vi "Error Channels Read Single.vi"(8 "error in":errorcluster, 9 "Channel Index":i32=1, 11 "Error Channels In":refnum<class "Error Channels.lvclass">) -> (0 "error out":errorcluster, 1 "Changed or First Call?":bool, 2 "Error Acknowledge Channels ACT":bool, 3 "Error Channels Out":refnum<class "Error Channels.lvclass">)   [LabVIEW 2023, in "Error Channels.lvclass"]
uses:
  Error Channels.lvclass
  Error Channels.lvclass/Error Channels.ctl
  <vilib>/ADAS Replay HIL/Channels/Tag Wrapper/Polymorphic/Read Channel (Boolean).vi
  fe5b2b55-f13d-4754-bc7f-45dbc12555c6.vi
  <vilib>/ADAS Replay HIL/Channels/Tag Wrapper/Polymorphic/Read Channel (Boolean).vi/b2f764de-0c1e-4784-a155-687fc995a684.vi
  <vilib>/ADAS Replay HIL/Channels/Tag Wrapper/Polymorphic/Read Channel (Boolean).vi/b2f764de-0c1e-4784-a155-687fc995a684.vi/c28b0ead-42ad-4072-80a2-aca7f2bd7ce3.vi
  <vilib>/ADAS Replay HIL/Channels/Tag Wrapper/Polymorphic/Read Channel (Boolean).vi/b2f764de-0c1e-4784-a155-687fc995a684.vi/219d0231-d98b-4193-b5cc-84f90e3c9091.vi
  <vilib>/ADAS Replay HIL/Channels/Tag Wrapper/Tag Wrapper.lvlib
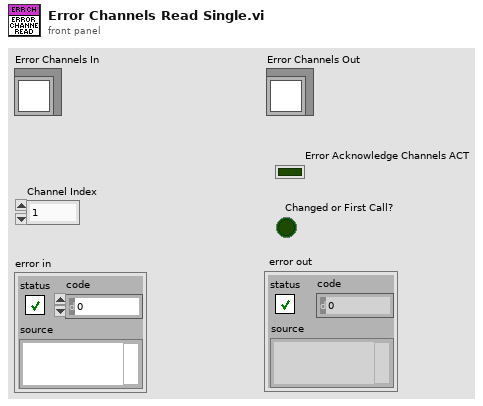
[diagram p1: front panel]
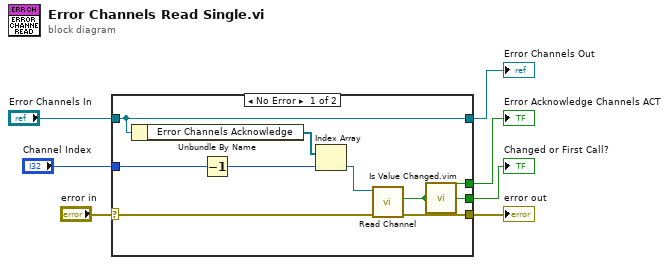
[diagram p0: block diagram]
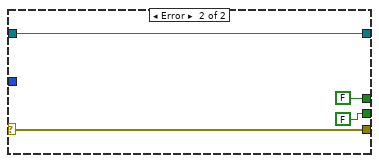
[diagram p2: hidden frame]
diagram:
  n1 = case shown="No Error" "error in" {
    selector: "error in" -> [w16 w20]
    tunnel: [w15 w20] -> w6
    tunnel: [w10 w19] -> w1
    tunnel: "Error Channels In" -> [w10 w19]
    tunnel: [w14 FALSE ("Value out")] -> w3
    tunnel: [w13 FALSE ("changed or first call?")] -> w5
    tunnel: "Channel Index" -> [w12 _]
    frame No Error {
      n2 = Unbundle By Name(w10) -> ("Error Channels Acknowledge"=w9:refnum<k21>[])
      n3 = Decrement(x=w12) -> (x-1=w11:i32)
      n4 = Index Array(array=w9, index=w11) -> (element=w8:refnum<k21>)
      n5 = call-poly <vilib>:"Read Channel.vi"("error in"=w16, "ADAS HIL Channel in"=w8) -> ("error out"=w15:errorcluster, "Value out"=w14:bool)  [unwired: 6 in, 2 out]
      n6 = call "Is Value Changed.vim"("value"=w14) -> ("changed or first call?"=w13:bool)
    }
    frame Error {
    }
  }
  "error out" <- w6
  "Changed or First Call?" <- w5
  "Error Acknowledge Channels ACT" <- w3
  "Error Channels Out" <- w1
